vi "Read Network Slave.vi"(8 "error in":errorcluster, 11 "Modbus slave in":refnum<class "Modbus Slave.lvclass">) -> (0 "error out":errorcluster, 2 "network slave":refnum<class "Network Slave.lvclass">, 3 "Modbus slave out":refnum<class "Modbus Slave.lvclass">)   [LabVIEW 2015, in "Modbus Library.lvlib" / "Modbus Slave.lvclass"]
doc: "This VI is an accessor for the <B>network slave</B> stored in the Modbus slave instance. This accessor can be used as a property node. This network slave is used by the Modbus instance to communicate on the physical bus."
uses:
  Modbus Slave.lvclass
  Network Protocol/Network Slave/Network Slave.lvclass
  Modbus Slave.lvclass/Modbus Slave.ctl
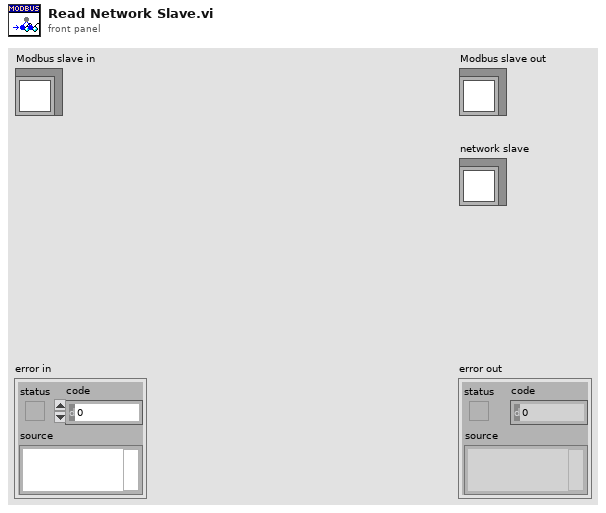
[diagram p1: front panel]
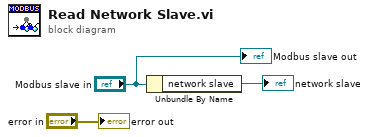
[diagram p0: block diagram]
diagram:
  n1 = Unbundle By Name("Modbus slave in") -> ("network slave"=→"network slave":refnum<class "Network Slave.lvclass">)
  "error out" <- "error in"
  "Modbus slave out" <- "Modbus slave in"
